vi "From Reference.vi"(1 "Transform Ref in":refnum<vi>) -> (0 "Transform out":refnum<class "Transform.lvclass">)   [LabVIEW 2022 SP3, in "Transform.lvclass"]
uses:
  Transform.lvclass
  Transform.lvclass/Transform.ctl
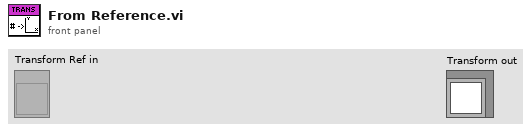
[diagram p1: front panel]
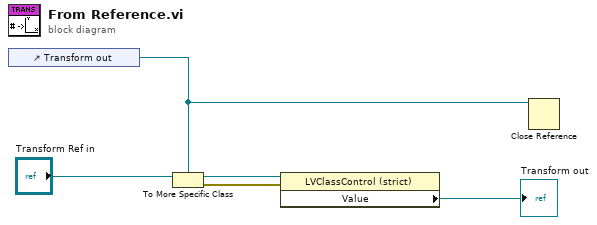
[diagram p0: block diagram]
diagram:
  n1 = control-ref of="Transform out"() -> (w2:refnum<vi>)
  n2 = To More Specific Class(target class=w2, reference="Transform Ref in") -> (specific class reference=w4:refnum<vi>, error out=w5:errorcluster)  [unwired: 1 in]
  n3 = property class="LVClassControl (strict)"(reference=w4, error in=w5) -> ("Value"=→"Transform out":refnum<class "Transform.lvclass">)  [unwired: 2 out]
  n4 = Close Reference(reference=w2) -> ()  [unwired: 1 in, 1 out]
